vi "Load Old Configurations.vi"() -> (0 "error out":errorcluster, 2 "Config Matches":bool)   [LabVIEW 2015, in "SystemLink Tag Module tests.lvlib"]
doc: "Test checks whether we are able to deserialize old configurations.\n\nTest should be updated for every configuration version bump."
uses:
  SystemLink Tag Module tests.lvlib
  module/configuration/SystemLink configuration.lvclass
  module/configuration/Data Tag Type.ctl
  <vilib>/NI/Tag Bus/tag/Data Type.ctl
  <vilib>/NI/Tag Bus Module Framework/channel/channel classification.ctl
  module/configuration/SystemLink configuration.lvclass/SystemLink configuration.ctl
  <vilib>/NI/Tag Bus Module Framework/channel/TBM channel.lvclass/TBM channel.ctl
  <vilib>/NI/Tag Bus/tag/tag descriptor.lvclass/tag descriptor.ctl
  module/configuration/Read Lines.vi
  <vilib>/NI/Tag Bus Module Framework/channel/TBM channel.lvclass
  <vilib>/NI/Tag Bus/tag/tag descriptor.lvclass
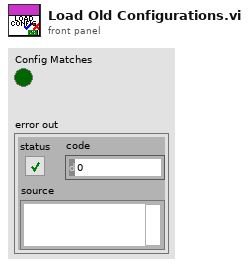
[diagram p1: front panel]
types:
  T1 = typedef "TBM channel.lvclass/channel classification.ctl" = enum16{"input data", "output data", "processing parameter", "processing result"}
  T2 = typedef "tag bus.lvlib/tag descriptor.lvclass/Data Type.ctl" = enum16{"Double", "Single", "I64", "I32", "I16", "I8", "U64", "U32", "U16", "U8", "Boolean", "String", "Array of Double", "Array of Single", "Array of I64", "Array of I32", "Array of I16", "Array of I8", "Array of U64", "Array of U32", "Array of U16", "Array of U8", "Array of Boolean", "Array of String"}
  T3 = typedef "SystemLink configuration.lvclass/Data Tag Type.ctl" = enum16{"Double", "Single", "I32", "I16", "I8", "U64", "U32", "U16", "U8", "Boolean", "String", "Timestamp"}
  T4 = typedef "SystemLink configuration.lvclass/Line.ctl" = cluster{"channel":refnum<class "TBM channel.lvclass">, "Data Tag Type":T3}
  T5 = cluster{"Data Tag Type":T3, "channel classification":T1, "data type":T2}
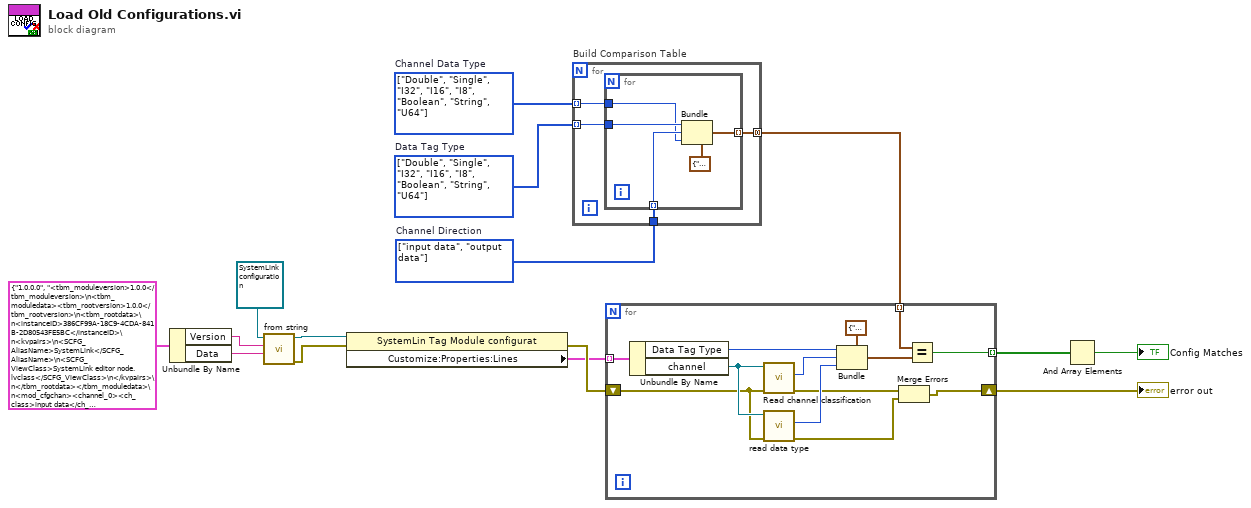
[diagram p0: block diagram]
diagram:
  w5 = T1[] [enum."input data", enum."output data"] items=["input data", "output data", "processing parameter", "processing result"]  # Channel Direction
  w7 = T2[] [enum."Double", enum."Single", enum."I32", enum."I16", enum."I8", enum."Boolean", enum."String", enum."U64"] items=["Double", "Single", "I64", "I32", "I16", "I8", "U64", "U32", "U16", "U8", "Boolean", "String", "Array of Double", "Array of Single", "Array of I64", "Array of I32", "Array of I16", "Array of I8", "Array of U64", "Array of U32", "Array of U16", "Array of U8", "Array of Boolean", "Array of String"]  # Channel Data Type
  w6 = T3[] [enum."Double", enum."Single", enum."I32", enum."I16", enum."I8", enum."Boolean", enum."String", enum."U64"] items=["Double", "Single", "I32", "I16", "I8", "U64", "U32", "U16", "U8", "Boolean", "String", "Timestamp"]  # Data Tag Type
  n1 = Unbundle By Name(cluster{"Version":string, "Data":string} {"Version"="1.0.0.0", "Data"="<tbm_moduleversion>1.0.0</tbm_moduleversion>\n<tbm_moduledata><tbm_rootversion>1.0.0</tbm_rootversion>\n<tbm_rootdata>\n<instanceID>386CF99A-18C9-4CDA-841B-2D80543FE5BC</instanceID>\n<kvpairs>\n<SCFG_AliasName>SystemLink</SCFG_AliasName>\n<SCFG_ViewClass>SystemLink editor node.lvclass</SCFG_ViewClass>\n</kvpairs>\n</tbm_rootdata></tbm_moduledata>\n<mod_cfgchan><channel_0><ch_class>input data</ch_class><default></default><meta></meta><ch_type>Double</ch_type><ch_version>1.0.0</ch_version></channel_0><channel_1><ch_class>output data</ch_class><default></default><meta></meta><ch_type>Double</ch_type><ch_version>1.0.0</ch_version></channel_1><channel_2><ch_class>input data</ch_class><default></default><meta></meta><ch_type>Single</ch_type><ch_version>1.0.0</ch_version></channel_2><channel_3><ch_class>output data</ch_class><default></default><meta></meta><ch_type>Single</ch_type><ch_version>1.0.0</ch_version></channel_3><channel_4><ch_class>input data</ch_class><default></default><meta></meta><ch_type>I32</ch_type><ch_version>1.0.0</ch_version></channel_4><channel_5><ch_class>output data</ch_class><default></default><meta></meta><ch_type>I32</ch_type><ch_version>1.0.0</ch_version></channel_5><channel_6><ch_class>input data</ch_class><default></default><meta></meta><ch_type>I16</ch_type><ch_version>1.0.0</ch_version></channel_6><channel_7><ch_class>output data</ch_class><default></default><meta></meta><ch_type>I16</ch_type><ch_version>1.0.0</ch_version></channel_7><channel_8><ch_class>input data</ch_class><default></default><meta></meta><ch_type>I8</ch_type><ch_version>1.0.0</ch_version></channel_8><channel_9><ch_class>output data</ch_class><default></default><meta></meta><ch_type>I8</ch_type><ch_version>1.0.0</ch_version></channel_9><channel_10><ch_class>input data</ch_class><default></default><meta></meta><ch_type>Boolean</ch_type><ch_version>1.0.0</ch_version></channel_10><channel_11><ch_class>output data</ch_class><default></default><meta></meta><ch_type>Boolean</ch_type><ch_version>1.0.0</ch_version></channel_11><channel_12><ch_class>input data</ch_class><default></default><meta></meta><ch_type>String</ch_type><ch_version>1.0.0</ch_version></channel_12><channel_13><ch_class>output data</ch_class><default></default><meta></meta><ch_type>String</ch_type><ch_version>1.0.0</ch_version></channel_13><channel_14><ch_class>input data</ch_class><default></default><meta></meta><ch_type>U64</ch_type><ch_version>1.0.0</ch_version></channel_14><channel_15><ch_class>output data</ch_class><default></default><meta></meta><ch_type>U64</ch_type><ch_version>1.0.0</ch_version></channel_15></mod_cfgchan>"}) -> ("Version"=w14:string, "Data"=w13:string)
  n2 = call-dynamic "from string.vi"("data"=w13, "version"=w14, "SystemLin Tag Module configuration in"=refnum<class "SystemLink configuration.lvclass"> refnum ("SystemLin Tag Module configuration")) -> ("error out"=w10:errorcluster, "SystemLin Tag Module configuration out"=w11:refnum<class "SystemLink configuration.lvclass">)  [unwired: 7 in]
  n3 = property class="SystemLin Tag Module configurat"(reference=w11, error in=w10) -> (error out=w9:errorcluster, "Customize:Properties:Lines"=w8:T4[])  [unwired: 1 out]
  n4 = for "Build Comparison Table" {
    tunnel: w7 -> [w18] mode=indexing
    tunnel: w6 -> [w17] mode=indexing
    tunnel: w5 -> [w19]
    tunnel: [w16] -> w4 mode=concatenating
    n5 = for {
      tunnel: w19 -> [w22] mode=indexing
      tunnel: w18 -> [w21]
      tunnel: w17 -> [w23]
      tunnel: [w20] -> w16 mode=indexing
      n6 = Bundle(cluster=T5 {"Data Tag Type"=enum."Double", "channel classification"=enum."input data", "data type"=enum."Double"}, "Data Tag Type"=w23, "channel classification"=w22, "data type"=w21) -> (w20:T5)
    }
  }
  n7 = for {
    tunnel: w8 -> [w37] mode=indexing
    shift-right: [w25] -> w3
    shift-left: w9 -> [w35]
    tunnel: w4 -> [w30] mode=indexing
    tunnel: [w28] -> w2 mode=indexing
    n8 = Unbundle By Name(w37) -> ("Data Tag Type"=w33:T3, "channel"=w36:refnum<class "TBM channel.lvclass">)
    n9 = call <vilib>:"Read channel classification.vi"("error in"=w35, "channel in"=w36) -> ("error out"=w27:errorcluster, "channel classification"=w32:T1)  [unwired: 7 in, 1 out]
    n10 = call <vilib>:"read data type.vi"("error in"=w35, "system tag in"=w36) -> ("error out"=w26:errorcluster, "data type"=w31:T2)  [unwired: 7 in, 1 out]
    n11 = Bundle(cluster=T5 {"Data Tag Type"=enum."Double", "channel classification"=enum."input data", "data type"=enum."Double"}, "Data Tag Type"=w33, "channel classification"=w32, "data type"=w31) -> (w29:T5)
    n12 = Merge Errors(w27, w26) -> (w25:errorcluster)
    n13 = Equal?(x=w30, y=w29) -> (x = y?=w28:bool)
  }
  "error out" <- w3
  n14 = And Array Elements(Boolean array=w2) -> (logical AND=→"Config Matches":bool)
